vi "test Empty File Part Results In Empty Path.vi"(8 "error in (no error)":errorcluster, 11 "TestCase in":refnum<class "Build Linux Log File Path.lvclass">) -> (0 "error out":errorcluster, 3 "TestCase out":refnum<class "Build Linux Log File Path.lvclass">)   [LabVIEW 2020, in "Build Linux Log File Path.lvclass"]
uses:
  Build Linux Log File Path.lvclass
  <vilib>/addons/_JKI Toolkits/VI Tester/TestCase.llb/TestCase.lvclass
  C:/Program Files (x86)/National Instruments/LabVIEW 2020/vi.lib/addons/_JKI Toolkits/VI Tester/TestCase.llb/TestCase.lvclass
  C:/Dev/GitHub/niveristand-ballard-arinc429-custom-device/Source/Custom Device Support/Tests/Unit/Shared/test Build Linux Log File Path/Build Linux Log File Path.lvclass
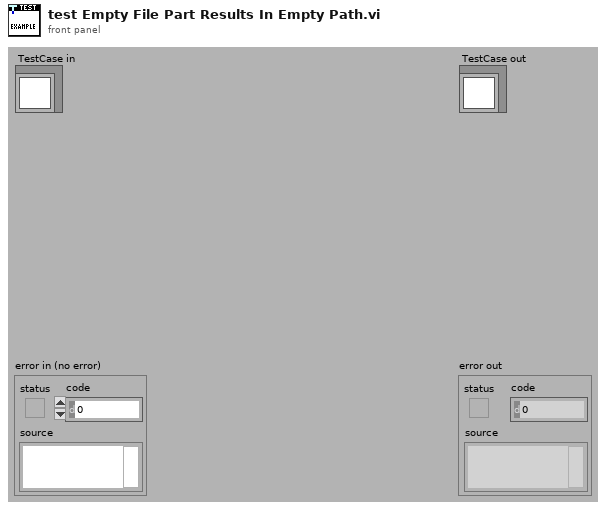
[diagram p1: front panel]
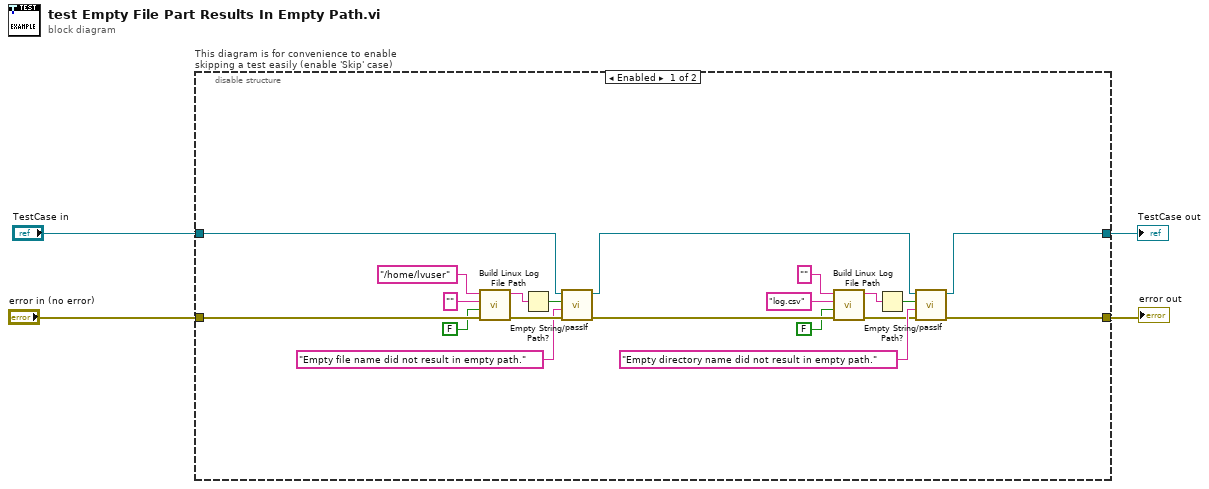
[diagram p0: block diagram]
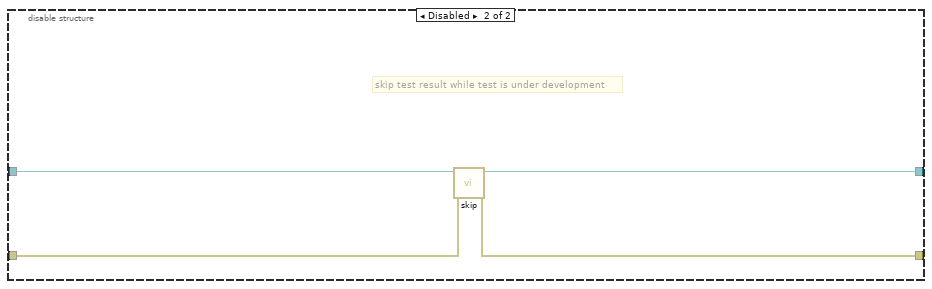
[diagram p2: hidden frame]
diagram:
  n1 = disable-structure "This diagram is for convenience to enable skipping a test easily (enable 'Skip' case)" shown="Enabled" {
    disable-tunnel: "TestCase in" -> [w22 w28]
    disable-tunnel: [w6 w26] -> w1
    disable-tunnel: [w5 w27] -> w3
    disable-tunnel: "error in (no error)" -> [w23 w25]
    frame Enabled {
      n2 = call "Build Linux Log File Path.vi"("error in (no error)"=w23, "Timestamp"=FALSE, "Name"="", "Log File Directory"="/home/lvuser") -> ("error out"=w20:errorcluster, "Log File Path"=w19:string)  [unwired: 6 in]
      n3 = Empty String/Path?(string/path=w19) -> (empty?=w21:bool)
      n4 = call-dynamic "passIf.vi"("error in (no error)"=w20, "message (\"\")"="Empty file name did not result in empty path." ("message (\"\")"), "pass"=w21, "TestCase in"=w22) -> ("error out"=w24:errorcluster, "TestCase out"=w7:refnum<class "Build Linux Log File Path.lvclass">)  [unwired: 6 in]
      n5 = call "Build Linux Log File Path.vi"("error in (no error)"=w24, "Timestamp"=FALSE, "Name"="log.csv", "Log File Directory"="") -> ("error out"=w9:errorcluster, "Log File Path"=w10:string)  [unwired: 6 in]
      n6 = Empty String/Path?(string/path=w10) -> (empty?=w8:bool)
      n7 = call-dynamic "passIf.vi"("error in (no error)"=w9, "message (\"\")"="Empty directory name did not result in empty path." ("message (\"\")"), "pass"=w8, "TestCase in"=w7) -> ("error out"=w5:errorcluster, "TestCase out"=w6:refnum<class "Build Linux Log File Path.lvclass">)  [unwired: 6 in]
    }
    frame Disabled {
      # "skip test result while test is under development"
      n8 = call <vilib>:"skip.vi"("error in (no error)"=w25, "TestCase in"=w28) -> ("error out"=w27:errorcluster, "TestCase in"=w26:refnum<class "Build Linux Log File Path.lvclass">)  [unwired: 8 in]
    }
  }
  "error out" <- w3
  "TestCase out" <- w1
